vi "NT Add ValueListener.vi"(10 "poller in":u32, 11 "listener info":T2 {"NT_Type" items=["NT_Unassigned"=0, "NT_Boolean"=1, "NT_Double"=2, "NT_String"=4, "NT_Raw"=8, "NT_BooleanArray"=16, "NT_DoubleArray"=32, "NT_StringArray"=64, "NT_RPC"=128, "NT_Integer"=256, "NT_Float"=512, "NT_IntegerArray"=1024, "NT_FloatArray"=2048]}) -> (2 "poller out":u32, 3 "return type":u32)   [LabVIEW 2025]
uses:
  <vilib>/Rock Robotics/Network Tables/NT Datatype.ctl
  <vilib>/Rock Robotics/Network Tables/NT SubscribeOptions.ctl
  ntcoreffi.dll
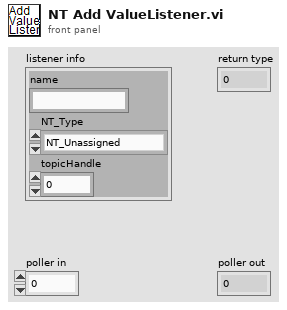
[diagram p1: front panel]
types:
  T1 = typedef "NT Datatype.ctl" = u32
  T2 = cluster{"name":string, "NT_Type":T1, "topicHandle":u32}
  T3 = typedef "NT SubscribeOptions.ctl" = cluster{"Send All":bool, "Keep Duplicates":bool, "rate (hz)":u64}
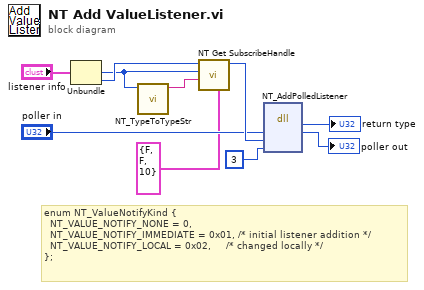
[diagram p0: block diagram]
diagram:
  # "enum NT_ValueNotifyKind {\n  NT_VALUE_NOTIFY_NONE = 0,\n  NT_VALUE_NOTIFY_IMMEDIATE = 0x01, /* initial listener addition */\n  NT_VALUE_NOTIFY_LOCAL = 0x02,     /* changed locally */\n};"
  n1 = Unbundle("listener info") -> ("NT_Type"=w9:T1, "topicHandle"=w10:u32)  [unwired: 1 out]
  n2 = call <vilib>:"NT_TypeToTypeStr.vi"("type"=w9) -> ("typeStr"=w8:string)  [unwired: 10 in]
  n3 = call <vilib>:"NT Get SubscribeHandle.vi"("options"=T3 {"Send All"=FALSE, "Keep Duplicates"=FALSE, "rate (hz)"=10}, "description"=w8, "NT_Type"=w9, "topicHandle"=w10) -> ("subscribeHandle"=w4:u32)  [unwired: 6 in, 1 out]
  n4 = dll-call lib="ntcoreffi.*" fn="NT_AddPolledListener"("poller"="poller in", "sub"=w4, "flags"=u32 3 ("Flags")) -> ("return type"=→"return type":u32, "poller"=→"poller out":u32)  [unwired: 5 in, 2 out]
